vi "Load EDS.vi"(8 "error in":errorcluster, 10 "EDS File Path":path, 11 "Interactor in":refnum<class "Interactor.lvclass">) -> (0 "error out":errorcluster, 3 "Interactor out":refnum<class "Interactor.lvclass">)   [LabVIEW 2024, in "Interactor.lvlib" / "Interactor.lvclass"]
uses:
  Interactor.lvclass
  EDS-File-Viewer/Core/EDS/EDS.lvclass
  EDS-File-Viewer/Core/EDS/EDS.lvclass/EDS.ctl
  Interactor.lvclass/Interactor.ctl
  Object Dictionary UI Messages/Populate OD Msg/Populate OD Msg.lvclass/Populate OD Msg.ctl
  <vilib>/ActorFramework/Message Enqueuer/Message Enqueuer.lvclass/Message Enqueuer.ctl
  Example/Home Messages/EDS File Loaded Msg/EDS File Loaded Msg.lvclass/EDS File Loaded Msg.ctl
  <vilib>/ActorFramework/Message Enqueuer/Enqueue.vi
  Object Dictionary UI Messages/Populate OD Msg/Populate OD Msg.lvclass
  C:/Program Files/National Instruments/LabVIEW 2024/vi.lib/ActorFramework/Message/Message.lvclass
  Example/Home Messages/EDS File Loaded Msg/EDS File Loaded Msg.lvclass
  <vilib>/Utility/LVClass/Get LV Class Name.vi
  <resource>/AFDebug/Generate Trace for Message.vi
  <vilib>/ActorFramework/Message Priority Queue/Priority Enqueue.vi
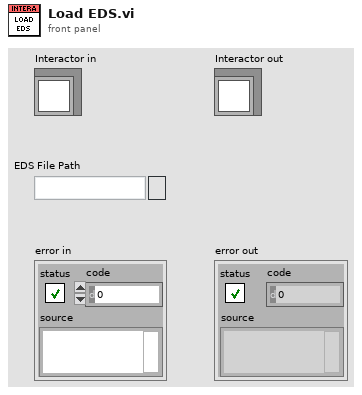
[diagram p1: front panel]
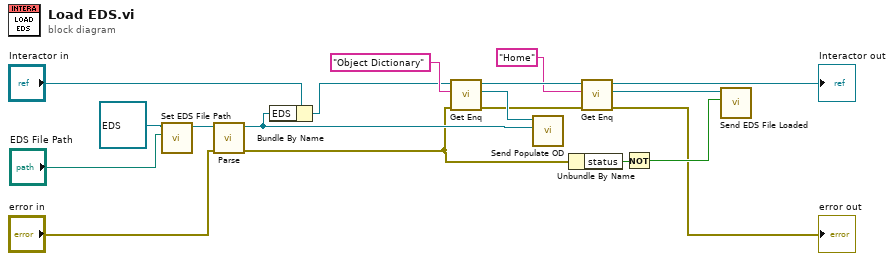
[diagram p0: block diagram]
diagram:
  n1 = call "Set EDS File Path.vi"("EDS File Path"="EDS File Path", "EDS in"=refnum<class "EDS.lvclass"> refnum) -> ("EDS out"=w16:refnum<class "EDS.lvclass">)  [unwired: 9 in]
  n2 = call "Parse.vi"("error in"="error in", "EDS in"=w16) -> ("error out"=w4:errorcluster, "EDS out"=w11:refnum<class "EDS.lvclass">)  [unwired: 8 in]
  n3 = Bundle By Name(cluster="Interactor in", "EDS"=w11) -> (w10:refnum<class "Interactor.lvclass">)
  n4 = call "Get Enq.vi"("error in"=w4, "Ident"="Object Dictionary", "Interactor in"=w10) -> ("error out"=w7:errorcluster, "Enq"=w13:refnum<class "Message Enqueuer.lvclass">, "Interactor out"=w18:refnum<class "Interactor.lvclass">)  [unwired: 6 in]
  n5 = call "Send Populate OD.vi"("EDS"=w11, "Message Enqueuer"=w13) -> ()  [unwired: 8 in, 2 out]
  n6 = Unbundle By Name(w4) -> ("status"=w3:bool)
  n7 = call "Get Enq.vi"("error in"=w7, "Ident"="Home", "Interactor in"=w18) -> ("error out"=→"error out":errorcluster, "Enq"=w5:refnum<class "Message Enqueuer.lvclass">, "Interactor out"=→"Interactor out":refnum<class "Interactor.lvclass">)  [unwired: 6 in]
  n8 = Not(x=w3) -> (.not. x?=w2:bool)
  n9 = call "Send EDS File Loaded.vi"("Valid?"=w2, "Message Enqueuer"=w5) -> ()  [unwired: 8 in, 2 out]
